vi "Alarm Value Check.vi"(8 "error in (no error)":errorcluster, 10 "Value":dbl, 11 "HK Alarms in":refnum<class "HK Alarms.lvclass">) -> (0 "error out":errorcluster, 2 "Alarm Status":T1, 3 "HK Alarms out":refnum<class "HK Alarms.lvclass">)   [LabVIEW 2024, in "HK Alarms.lvclass"]
uses:
  HK Alarms.lvclass
  HK Alarm enum Status.ctl
  HK Alarms.lvclass/HK Alarms.ctl
  HK Item/HK Item.lvclass
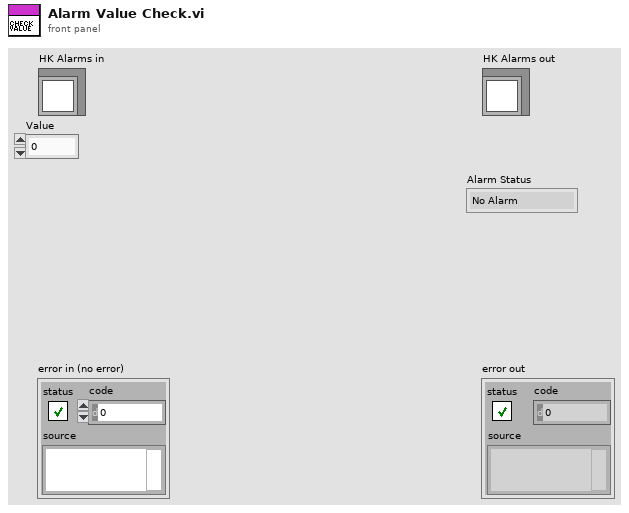
[diagram p1: front panel]
types:
  T1 = typedef "HK Item.lvclass/HK Alarm enum Status.ctl" = enum16{"No Alarm", "Red Low", "Red High", "Yellow Low", "Yellow High"}
  T2 = typedef "HK Item.lvclass/HK Channel Settings Alarms.ctl" = cluster{"Enabled":bool, "Deadband":i32, "Action":T3}
  T3 = typedef "HK Item.lvclass/HK Alarm enum Action.ctl" = enum16{"Light", "Message", "Safe"}
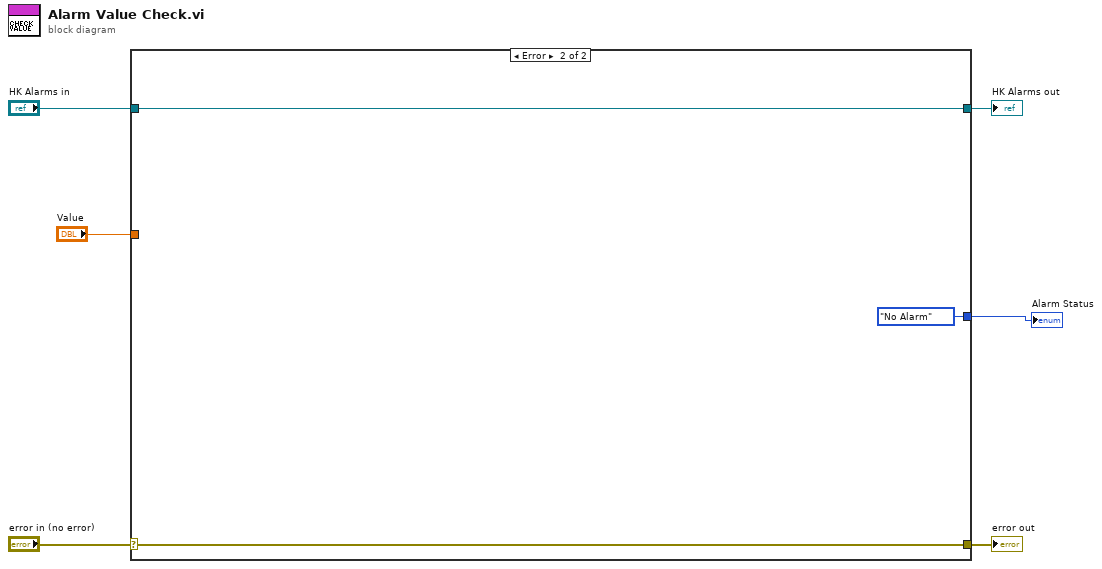
[diagram p0: block diagram]
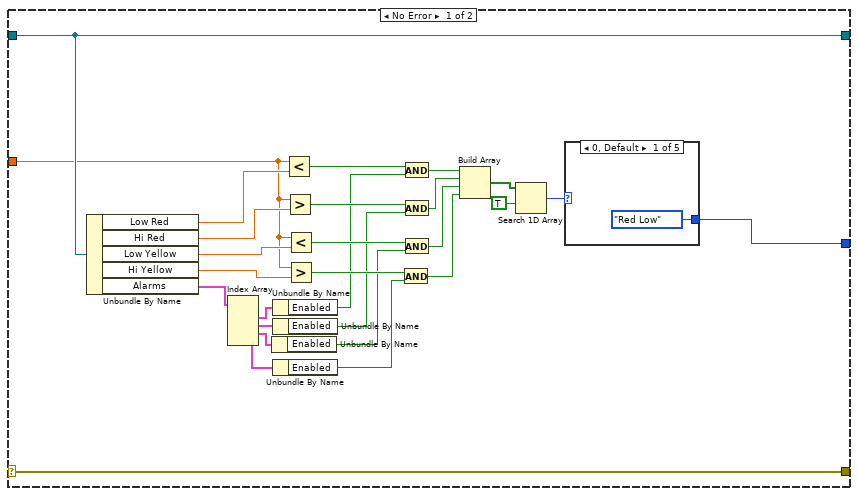
[diagram p2: hidden frame]
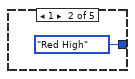
[diagram p3: hidden frame]
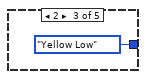
[diagram p4: hidden frame]
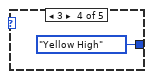
[diagram p5: hidden frame]
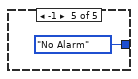
[diagram p6: hidden frame]
diagram:
  n1 = case shown="Error" "error in (no error)" {
    selector: "error in (no error)" -> [w34 w42]
    tunnel: [w34 w42] -> w5
    tunnel: [w9 w41] -> w3
    tunnel: "HK Alarms in" -> [w9 w41]
    tunnel: "Value" -> [w8 _]
    tunnel: [w7 HK_Alarm_enum_Status."No Alarm"] -> w1
    frame No Error {
      n2 = Unbundle By Name(w9) -> ("Low Red"=w33:dbl, "Hi Red"=w32:dbl, "Low Yellow"=w31:dbl, "Hi Yellow"=w30:dbl, "Alarms"=w25:T2[])
      n3 = Index Array(array=w25) -> (element #1=w24:T2, element #2=w23:T2, element #3=w22:T2, element #4=w21:T2)  [unwired: 4 in]
      n4 = Unbundle By Name(w22) -> ("Enabled"=w18:bool)
      n5 = Unbundle By Name(w24) -> ("Enabled"=w12:bool)
      n6 = Unbundle By Name(w23) -> ("Enabled"=w15:bool)
      n7 = Unbundle By Name(w21) -> ("Enabled"=w19:bool)
      n8 = Less?(x=w8, y=w33) -> (x < y?=w11:bool)
      n9 = Greater?(x=w8, y=w32) -> (0:w14:bool)
      n10 = Less?(x=w8, y=w31) -> (x < y?=w17:bool)
      n11 = Greater?(x=w8, y=w30) -> (0:w29:bool)
      n12 = And(x=w29, y=w19) -> (x .and. y?=w20:bool)
      n13 = And(x=w11, y=w12) -> (x .and. y?=w10:bool)
      n14 = And(x=w14, y=w15) -> (x .and. y?=w13:bool)
      n15 = And(x=w17, y=w18) -> (x .and. y?=w16:bool)
      n16 = Build Array(w10, w13, w16, w20) -> (w28:bool[])
      n17 = Search 1D Array(1D array=w28, element=TRUE) -> (index of element=w26:i32)  [unwired: 1 in]
      n18 = case shown="0, Default" w26 {
        tunnel: [HK_Alarm_enum_Status."Red Low" HK_Alarm_enum_Status."Red High" HK_Alarm_enum_Status."Yellow Low" HK_Alarm_enum_Status."Yellow High" HK_Alarm_enum_Status."No Alarm"] -> w7
        frame 0, Default {
        }
        frame 1 {
        }
        frame 2 {
        }
        frame 3 {
        }
        frame -1 {
        }
      }
    }
    frame Error {
    }
  }
  "error out" <- w5
  "HK Alarms out" <- w3
  "Alarm Status" <- w1
